vi "RESTful Get VI Parameter Info.vi"(8 "error in (no error)":errorcluster, 10 "control name prefix":string, 11 "Variant":variant) -> (0 "error out":errorcluster, 1 "has sub elements?":bool, 2 "Terminal Info Summary":T1, 3 "Elements":variant[](array[variant]), 4 "element control name prefix":string)   [LabVIEW 2020]
uses:
  <vilib>/AppBuilder/Engine/RESTful INI Generator/RESTful VI Terminal Info Summary.ctl
  <resource>/Framework/Providers/Common/provcom_StringGlobals.vi
  <vilib>/Utility/VariantDataType/VariantType.lvlib
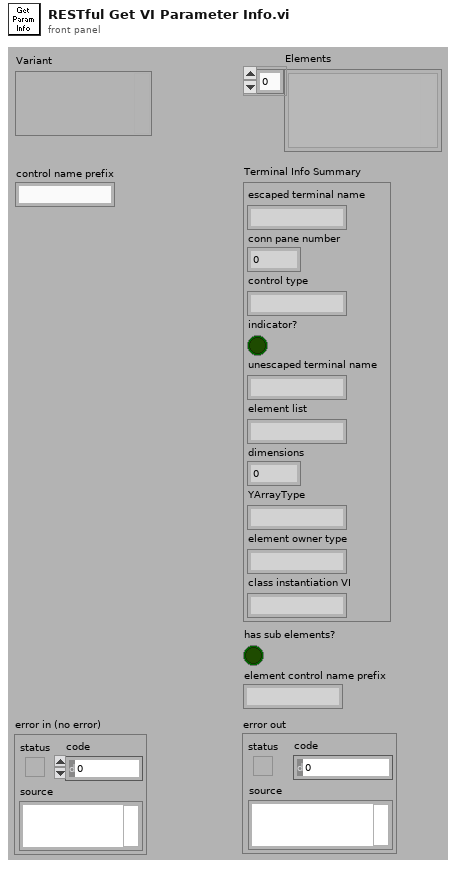
[diagram p1: front panel]
types:
  T1 = typedef "RESTful VI Terminal Info Summary.ctl" = cluster{"escaped terminal name":string, "conn pane number":i32, "control type":string, "indicator?":bool, "unescaped terminal name":string, "element list":string, "dimensions":u32, "YArrayType":string, "element owner type":string, "class instantiation VI":string}
  T2 = typedef "VariantType.lvlib/Type.ctl" = enum8{"Invalid Type", "Void", "I8", "I16", "I32", "I64", "U8", "U16", "U32", "U64", "Single Float", "Double Float", "Extended Float", "Single Complex", "Double Complex", "Extended Complex", "Enum U8", "Enum U16", "Enum U32", "Enum U64", "Single Float With Unit", "Double Float With Unit", "Extended Float With Unit", "Single Complex with Unit", "Double Complex with Unit", "Extended Complex with Unit", "Boolean", "String", "Path", "Picture", "Tag", "Array", "Cluster", "Variant", "LV Variant", "Waveform", "Timestamp", "Digital Waveform", "Digital Data", "ExpressData", "Refnum", "External Data", "VI", "Poly VI", "LabVIEW Class Instance", "Fixed Point"}
  T3 = typedef "VariantType.lvlib/TypedefInfo.ctl" = cluster{"Name":string, "Timestamp":u32}
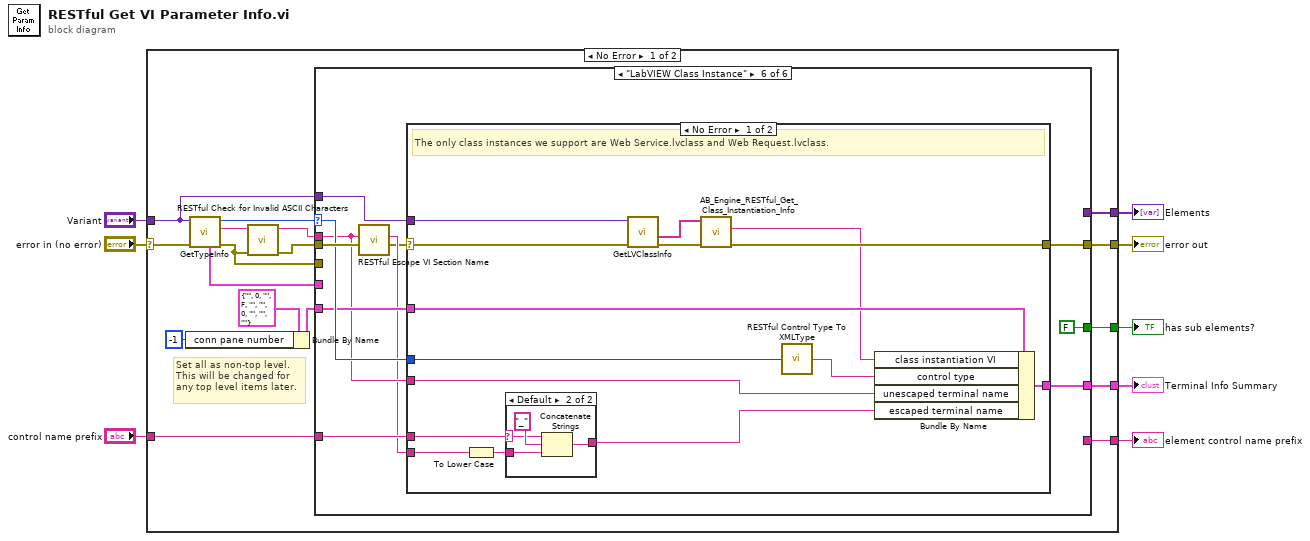
[diagram p0: block diagram]
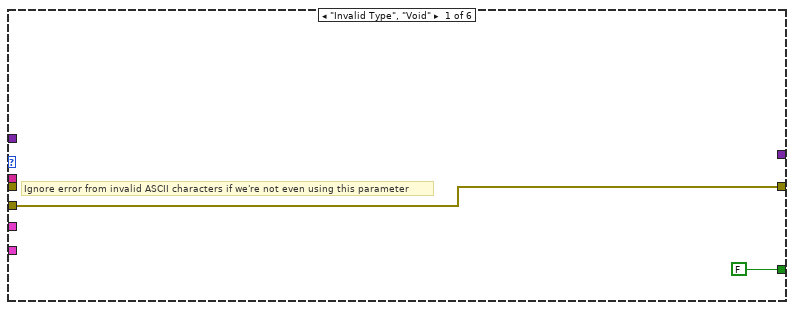
[diagram p2: hidden frame]
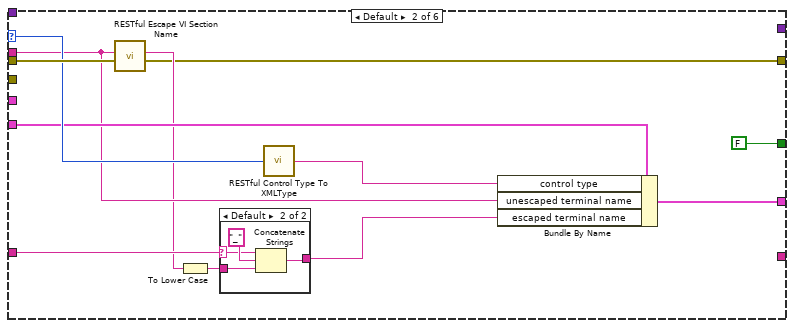
[diagram p3: hidden frame]
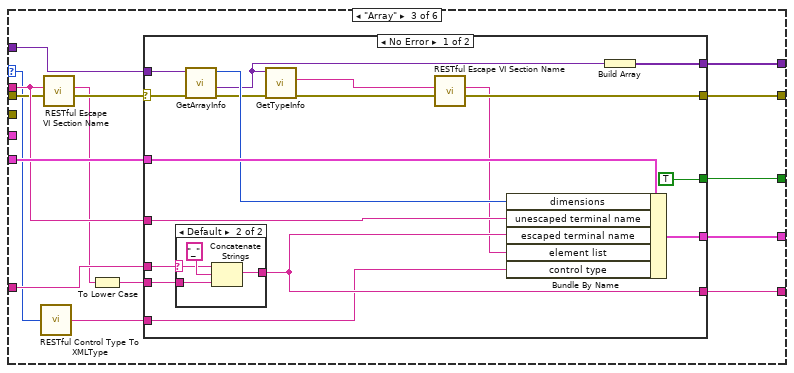
[diagram p5: hidden frame]
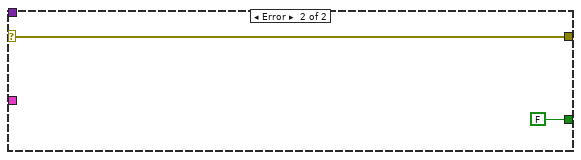
[diagram p7: hidden frame]
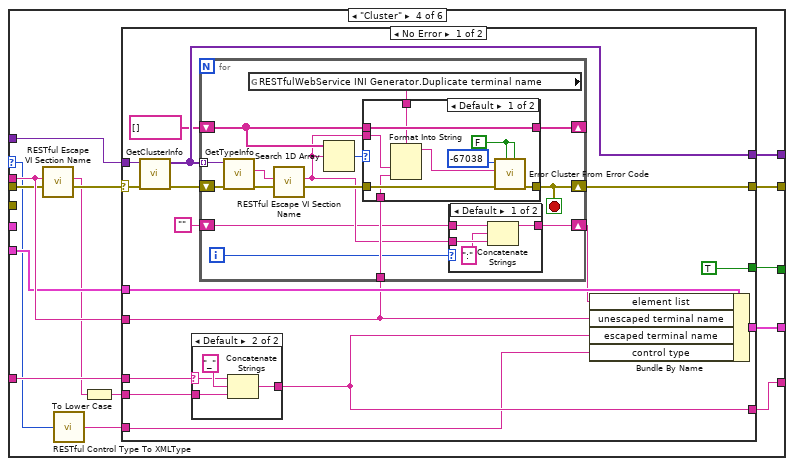
[diagram p8: hidden frame]
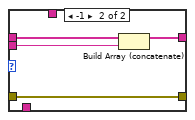
[diagram p10: hidden frame]
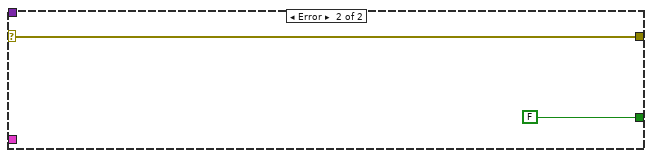
[diagram p12: hidden frame]
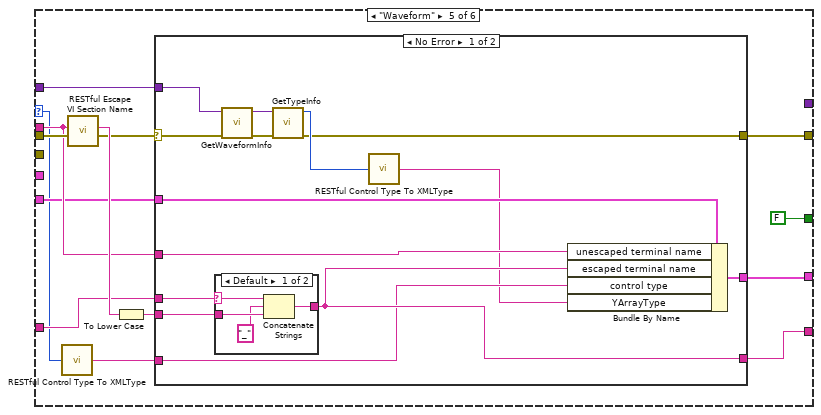
[diagram p13: hidden frame]
diagram:
  n1 = case shown="No Error" "error in (no error)" {
    selector: "error in (no error)" -> [w14 w222]
    tunnel: "Variant" -> [w24 _]
    tunnel: [w22 _] -> w7
    tunnel: [w21 w222] -> w6
    tunnel: [w20 _] -> w5
    tunnel: [w19 _] -> w4
    tunnel: "control name prefix" -> [w18 _]
    tunnel: [w17 _] -> w2
    frame No Error {
      # "Set all as non-top level.\nThis will be changed for\nany top level items later."
      n2 = Bundle By Name(cluster=T1 {"escaped terminal name"="", "conn pane number"=0, "control type"="", "indicator?"=FALSE, "unescaped terminal name"="", "element list"="", "dimensions"=0, "YArrayType"="", "element owner type"="", "class instantiation VI"=""} ("Terminal Info Summary"), "conn pane number"=-1) -> (w16:T1)
      n3 = call <vilib>:"GetTypeInfo.vi"("error in (no error)"=w14, "Variant"=w24) -> ("error out"=w10:errorcluster, "Name"=w12:string, "Type Enum"=w25:T2, "TypedefInfo"=w9:T3)  [unwired: 6 out]
      n4 = call <vilib>:"RESTful Check for Invalid ASCII Characters.vi"("error in (no error)"=w10, "Parameter Name"=w12) -> ("error out"=w13:errorcluster, "dup Parameter Name"=w11:string)  [unwired: 8 in]
      n5 = case shown="\"LabVIEW Class Instance\"" w25 {
        selector: w25 -> [_ w38 w47 w86 w159 w199]
        tunnel: w24 -> [_ _ w59 w98 w164 w190]
        tunnel: w13 -> [_ w39 w56 w96 w169 w200]
        tunnel: w11 -> [_ w32 w57 w97 w163 w194]
        tunnel: w16 -> [_ w35 w58 w95 w161 w197]
        tunnel: [_ w36 w54 w94 w162 w198] -> w22
        tunnel: [w26 w28 w53 w93 w156 w191] -> w21
        tunnel: [FALSE ("sub element") FALSE ("sub element") w52 w92 FALSE ("has sub elements? 2") FALSE ("sub element")] -> w20
        tunnel: [_ _ w45 w91 _ _] -> w19
        tunnel: w18 -> [_ w33 w51 w90 w166 w195]
        tunnel: [_ _ w50 w89 w160 _] -> w17
        tunnel: w10 -> [w26 _ _ _ _ _]
        tunnel: w9 -> [_ _ _ _ _ _]
        frame "Invalid Type", "Void" {
          # "Ignore error from invalid ASCII characters if we're not even using this parameter"
        }
        frame Default {
          n6 = call <vilib>:"RESTful Escape VI Section Name.vi"("error in"=w39, "Label.Text"=w32) -> ("error out"=w28:errorcluster, "result string"=w30:string)  [unwired: 8 out]
          n7 = To Lower Case(string=w30) -> (all lower case string=w29:string)
          n8 = case shown="Default" w33 {
            selector: w33 -> [_ w41]
            tunnel: [w40 w43] -> w31
            tunnel: w29 -> [w40 w42]
            frame "" {
            }
            frame Default {
              n9 = Concatenate Strings(w41, "_" ("string"), w42) -> (w43:string)
            }
          }
          n10 = call <vilib>:"RESTful Control Type To XMLType.vi"("Type Enum"=w38) -> ("Control Type XML"=w37:string)
          n11 = Bundle By Name(cluster=w35, "control type"=w37, "unescaped terminal name"=w32, "escaped terminal name"=w31) -> (w36:T1)
        }
        frame "Array" {
          n12 = call <vilib>:"RESTful Control Type To XMLType.vi"("Type Enum"=w47) -> ("Control Type XML"=w46:string)
          n13 = call <vilib>:"RESTful Escape VI Section Name.vi"("error in"=w56, "Label.Text"=w57) -> ("error out"=w55:errorcluster, "result string"=w48:string)  [unwired: 8 out]
          n14 = To Lower Case(string=w48) -> (all lower case string=w49:string)
          n15 = case shown="No Error" w55 {
            selector: w55 -> [w73 w84]
            tunnel: w59 -> [w77 _]
            tunnel: w58 -> [w76 _]
            tunnel: w57 -> [w74 _]
            tunnel: w49 -> [w68 _]
            tunnel: [w72 _] -> w54
            tunnel: [w62 w84] -> w53
            tunnel: [TRUE ("sub element") FALSE ("sub element")] -> w52
            tunnel: [w64 _] -> w45
            tunnel: w51 -> [w67 _]
            tunnel: [w69 _] -> w50
            tunnel: w46 -> [w66 _]
            frame No Error {
              n16 = case shown="Default" w67 {
                selector: w67 -> [_ w79]
                tunnel: [w78 w81] -> w69
                tunnel: w68 -> [w78 w80]
                frame "" {
                }
                frame Default {
                  n17 = Concatenate Strings(w79, "_" ("string"), w80) -> (w81:string)
                }
              }
              n18 = call <vilib>:"GetArrayInfo.vi"("error in (no error)"=w73, "Variant"=w77) -> ("error out"=w70:errorcluster, "ArrayElement"=w65:variant, "NDims"=w75:i32)  [unwired: 7 out]
              n19 = call <vilib>:"GetTypeInfo.vi"("error in (no error)"=w70, "Variant"=w65) -> ("error out"=w63:errorcluster, "Name"=w61:string)  [unwired: 8 out]
              n20 = call <vilib>:"RESTful Escape VI Section Name.vi"("error in"=w63, "Label.Text"=w61) -> ("error out"=w62:errorcluster, "result string"=w60:string)  [unwired: 8 out]
              n21 = Bundle By Name(cluster=w76, "dimensions"=w75, "unescaped terminal name"=w74, "escaped terminal name"=w69, "element list"=w60, "control type"=w66) -> (w72:T1)
              n22 = Build Array(w65) -> (w64:variant[])
            }
            frame Error {
            }
          }
        }
        frame "Cluster" {
          n23 = call <vilib>:"RESTful Escape VI Section Name.vi"("error in"=w96, "Label.Text"=w97) -> ("error out"=w99:errorcluster, "result string"=w88:string)  [unwired: 8 out]
          n24 = call <vilib>:"RESTful Control Type To XMLType.vi"("Type Enum"=w86) -> ("Control Type XML"=w85:string)
          n25 = To Lower Case(string=w88) -> (all lower case string=w87:string)
          n26 = case shown="No Error" w99 {
            selector: w99 -> [w113 w155]
            tunnel: w98 -> [w115 _]
            tunnel: w95 -> [w114 _]
            tunnel: w97 -> [w100 _]
            tunnel: w87 -> [w105 _]
            tunnel: [w112 _] -> w94
            tunnel: [w107 w155] -> w93
            tunnel: [TRUE ("sub element") FALSE ("sub element")] -> w92
            tunnel: [w102 _] -> w91
            tunnel: w90 -> [w106 _]
            tunnel: [w104 _] -> w89
            tunnel: w85 -> [w103 _]
            frame No Error {
              n27 = call <vilib>:"GetClusterInfo.vi"("error in (no error)"=w113, "Variant"=w115) -> ("error out"=w110:errorcluster, "Cluster Elements"=w102:variant[])  [unwired: 8 out]
              n28 = case shown="Default" w106 {
                selector: w106 -> [_ w117]
                tunnel: [w116 w119] -> w104
                tunnel: w105 -> [w116 w118]
                frame "" {
                }
                frame Default {
                  n29 = Concatenate Strings(w117, "_" ("string"), w118) -> (w119:string)
                }
              }
              n30 = for {
                tunnel: w102 -> [w134] mode=indexing
                shift-right: [w126] -> w107
                shift-left: w110 -> [w135]
                shift-right: [w133] -> w108
                shift-left: "" -> [w122]
                shift-right: [w128] -> _
                shift-left: string[] [] -> [w129]
                tunnel: w100 -> [w124]
                i -> [w121]
                stop <- w126 stop-if-true
                n31 = call <vilib>:"GetTypeInfo.vi"("error in (no error)"=w135, "Variant"=w134) -> ("error out"=w132:errorcluster, "Name"=w127:string)  [unwired: 8 out]
                n32 = global read "provcom_StringGlobals.vi" "RESTfulWebService INI Generator.Duplicate terminal name"() -> (w125:string)
                n33 = call <vilib>:"RESTful Escape VI Section Name.vi"("error in"=w132, "Label.Text"=w127) -> ("error out"=w130:errorcluster, "result string"=w123:string)  [unwired: 8 out]
                n34 = Search 1D Array(1D array=w129, element=w123) -> (index of element=w131:i32)  [unwired: 1 in]
                n35 = case shown="Default" w131 {
                  tunnel: w130 -> [w141 w145]
                  tunnel: w129 -> [w144 w148]
                  tunnel: [w144 w147] -> w128
                  tunnel: w123 -> [w137 w146]
                  tunnel: [w140 w145] -> w126
                  tunnel: w125 -> [w139 _]
                  tunnel: w124 -> [w136 _]
                  frame Default {
                    w142 = FALSE ("is warning? (False)")
                    n36 = Format Into String(format string=w139, w137, w136) -> (resulting string=w138:string)  [unwired: 2 in, 1 out]
                    n37 = call <vilib>:"Error Cluster From Error Code.vi"("is warning? (False)"=w142, "show call chain? (False)"=w142, "error in (no error)"=w141, "error message (\"\")"=w138, "error code (0)"=-67038) -> ("error out"=w140:errorcluster)  [unwired: 4 out]
                  }
                  frame -1 {
                    n38 = Build Array (concatenate)(w148, w146) -> (w147:string[])
                  }
                }
                n39 = case shown="Default" w121 {
                  tunnel: [w152 w153] -> w133
                  tunnel: w123 -> [w151 w153]
                  tunnel: w122 -> [w149 _]
                  frame Default {
                    n40 = Concatenate Strings(w149, ":" ("string"), w151) -> (w152:string)
                  }
                  frame 0 {
                  }
                }
              }
              n41 = Bundle By Name(cluster=w114, "element list"=w108, "unescaped terminal name"=w100, "escaped terminal name"=w104, "control type"=w103) -> (w112:T1)
            }
            frame Error {
            }
          }
        }
        frame "Waveform" {
          n42 = call <vilib>:"RESTful Control Type To XMLType.vi"("Type Enum"=w159) -> ("Control Type XML"=w158:string)
          n43 = call <vilib>:"RESTful Escape VI Section Name.vi"("error in"=w169, "Label.Text"=w163) -> ("error out"=w167:errorcluster, "result string"=w168:string)  [unwired: 8 out]
          n44 = To Lower Case(string=w168) -> (all lower case string=w165:string)
          n45 = case shown="No Error" w167 {
            selector: w167 -> [w181 w189]
            tunnel: w166 -> [w183 _]
            tunnel: w165 -> [w182 _]
            tunnel: w164 -> [w180 _]
            tunnel: w163 -> [w177 _]
            tunnel: [w176 _] -> w162
            tunnel: w161 -> [w175 _]
            tunnel: [w174 _] -> w160
            tunnel: w158 -> [w173 _]
            tunnel: [w170 w189] -> w156
            frame No Error {
              n46 = case shown="Default" w183 {
                selector: w183 -> [w186 _]
                tunnel: w182 -> [w187 w188]
                tunnel: [w184 w188] -> w174
                frame Default {
                  n47 = Concatenate Strings(w186, "_" ("string"), w187) -> (w184:string)
                }
                frame "" {
                }
              }
              n48 = call <vilib>:"GetWaveformInfo.vi"("error in (no error)"=w181, "Variant"=w180) -> ("error out"=w178:errorcluster, "YArrayType"=w179:variant)  [unwired: 8 out]
              n49 = call <vilib>:"GetTypeInfo.vi"("error in (no error)"=w178, "Variant"=w179) -> ("error out"=w170:errorcluster, "Type Enum"=w172:T2)  [unwired: 8 out]
              n50 = call <vilib>:"RESTful Control Type To XMLType.vi"("Type Enum"=w172) -> ("Control Type XML"=w171:string)
              n51 = Bundle By Name(cluster=w175, "unescaped terminal name"=w177, "escaped terminal name"=w174, "control type"=w173, "YArrayType"=w171) -> (w176:T1)
            }
            frame Error {
            }
          }
        }
        frame "LabVIEW Class Instance" {
          n52 = call <vilib>:"RESTful Escape VI Section Name.vi"("error in"=w200, "Label.Text"=w194) -> ("error out"=w192:errorcluster, "result string"=w193:string)  [unwired: 8 out]
          n53 = case shown="No Error" w192 {
            selector: w192 -> [w203 w221]
            tunnel: w199 -> [w207 _]
            tunnel: [w214 _] -> w198
            tunnel: w197 -> [w213 _]
            tunnel: w195 -> [w212 _]
            tunnel: w194 -> [w211 _]
            tunnel: w193 -> [w209 _]
            tunnel: [w206 w221] -> w191
            tunnel: w190 -> [w204 _]
            frame No Error {
              # "The only class instances we support are Web Service.lvclass and Web Request.lvclass."
              n54 = To Lower Case(string=w209) -> (all lower case string=w208:string)
              n55 = case shown="Default" w212 {
                selector: w212 -> [_ w217]
                tunnel: [w216 w219] -> w210
                tunnel: w208 -> [w216 w218]
                frame "" {
                }
                frame Default {
                  n56 = Concatenate Strings(w217, "_" ("string"), w218) -> (w219:string)
                }
              }
              n57 = call <vilib>:"GetLVClassInfo.vi"("error in (no error)"=w203, "Variant"=w204) -> ("error out"=w201:errorcluster, "Fully Qualified LV Class Name"=w202:string[])  [unwired: 7 in, 1 out]
              n58 = call <vilib>:"AB_Engine_RESTful_Get_Class_Instantiation_Info.vi"("error in (no error)"=w201, "fully qualified LV class name"=w202) -> ("error out"=w206:errorcluster, "qualified instantiation VI name"=w205:string)  [unwired: 7 in, 1 out]
              n59 = call <vilib>:"RESTful Control Type To XMLType.vi"("Type Enum"=w207) -> ("Control Type XML"=w215:string)
              n60 = Bundle By Name(cluster=w213, "class instantiation VI"=w205, "control type"=w215, "unescaped terminal name"=w211, "escaped terminal name"=w210) -> (w214:T1)
            }
            frame Error {
            }
          }
        }
      }
    }
    frame Error {
    }
  }
  "Terminal Info Summary" <- w7
  "error out" <- w6
  "has sub elements?" <- w5
  "Elements" <- w4
  "element control name prefix" <- w2
